vi "LeadLag_Execute.vi"(6 "Time (Secs)":dbl=-1.0, 8 "Lag Time Const (Sec)":dbl, 9 "Lead Time Const (Sec)":dbl, 10 "Enable":bool=TRUE, 11 "Input":dbl) -> (3 "Output":dbl)   [LabVIEW 2019, in "Trajectory_Library.lvlib"]
uses:
  <vilib>/Rock Robotics/WPI/ThirdParty/JAS_Junk/TrajLib/Trajectory_Library.lvlib
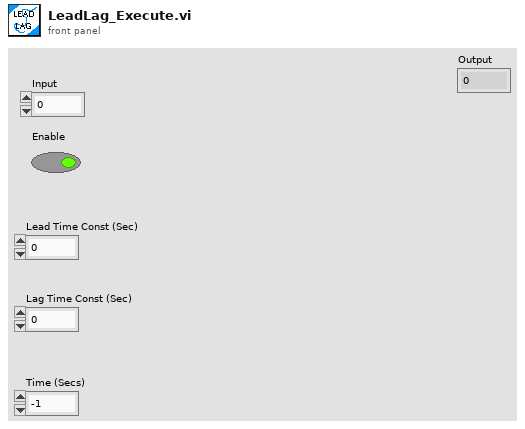
[diagram p1: front panel]
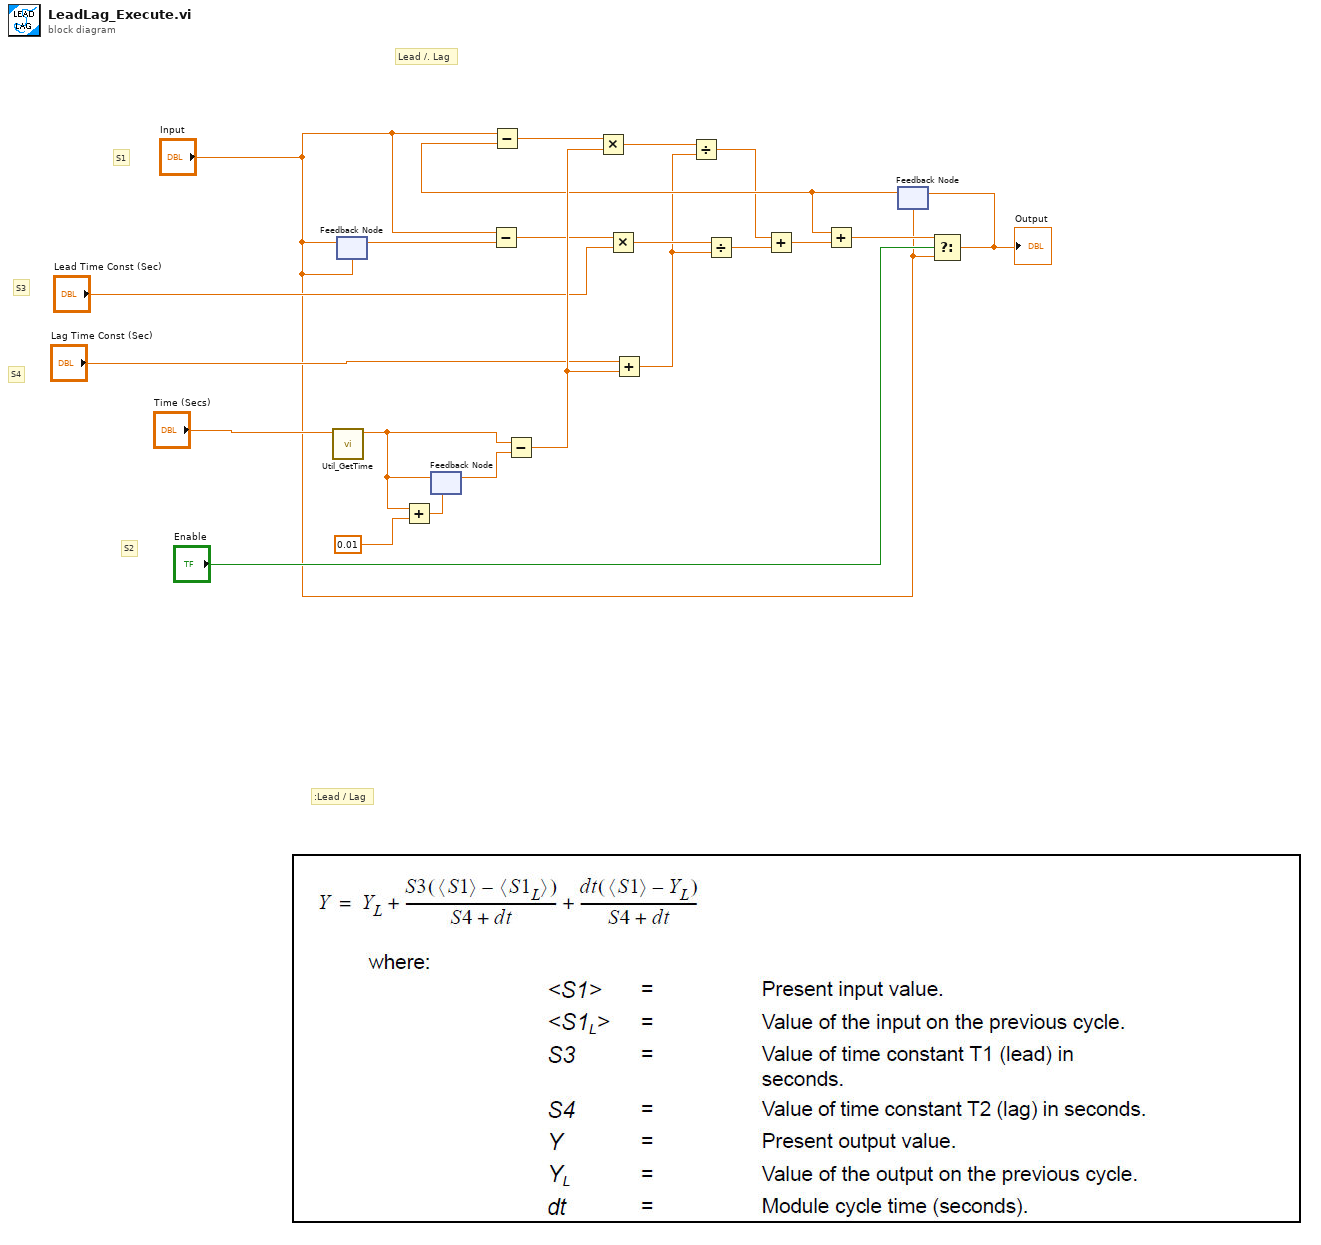
[diagram p0: block diagram]
diagram:
  # "Lead /. Lag"
  # "S2"
  # "S4"
  # "S3"
  # "S1"
  # ":Lead / Lag"
  n1 = call <vilib>:"Util_GetTime.vi"("Pass_Through_Time"="Time (Secs)") -> ("FPGA_Time_Seconds"=w16:dbl)  [unwired: 9 in, 1 out]
  n2 = feedback-in #1("Input") -> ()
  n3 = feedback #1("Input") -> (w9:dbl)
  n4 = Add(x=w16, y=0.01) -> (x+y=w20:dbl)
  n5 = feedback-in #2(w16) -> ()
  n6 = feedback #2(w20) -> (w22:dbl)
  n7 = Subtract(x="Input", y=w9) -> (x-y=w8:dbl)
  n8 = Subtract(x=w16, y=w22) -> (x-y=w19:dbl)
  n9 = Multiply(x=w8, y="Lead Time Const (Sec)") -> (x*y=w7:dbl)
  n10 = Add(x="Lag Time Const (Sec)", y=w19) -> (x+y=w4:dbl)
  n11 = Divide(x=w7, y=w4) -> (x/y=w2:dbl)
  n12 = feedback #3("Input") -> (w11:dbl)
  n13 = Subtract(x="Input", y=w11) -> (x-y=w6:dbl)
  n14 = Multiply(x=w6, y=w19) -> (x*y=w5:dbl)
  n15 = Divide(x=w5, y=w4) -> (x/y=w3:dbl)
  n16 = Add(x=w3, y=w2) -> (x+y=w1:dbl)
  n17 = Add(x=w11, y=w1) -> (x+y=w13:dbl)
  n18 = Select(t=w13, s="Enable", f="Input") -> (s? t:f=w12:dbl)
  "Output" <- w12
  n19 = feedback-in #3(w12) -> ()
